vi "CODMn报警信息存储.vi"(8 "error in (no error)":errorcluster, 11 "data in":T1) -> (0 "error out":errorcluster)   [LabVIEW 2016, in "斯坦道CODMn.lvlib"]
uses:
  <vilib>/addons/database/Auxilliary.llb/DB Tools Transaction.ctl
  <vilib>/addons/database/Auxilliary.llb/DB Tools Isolation Level.ctl
  <vilib>/addons/database/Auxilliary.llb/DB Tools Column Info.ctl
  <vilib>/addons/database/Auxilliary.llb/DB Tools DataTypes.ctl
  <vilib>/addons/database/Auxilliary.llb/DB Tools Parameter Info.ctl
  <vilib>/addons/database/Auxilliary.llb/DB Tools Parameter Dir.ctl
  <vilib>/addons/database/Connection.llb/DB Tools Open Connec (String).vi
  <vilib>/addons/database/Connection.llb/Conn Transaction.vi
  <vilib>/addons/database/Connection.llb/Conn Execute.vi
  <vilib>/addons/database/Recordset.llb/Rec Destroy - Connection.vi
  <vilib>/addons/database/Command.llb/Cmd Set Parameter Value (C).vi
  <vilib>/addons/database/Auxilliary.llb/DB Tools Format Datetime String (Time Stamp).vi
  <vilib>/addons/database/Command.llb/Cmd Execute.vi
  <vilib>/addons/database/Recordset.llb/Rec Destroy - Command.vi
  <vilib>/addons/database/Command.llb/Cmd Delete.vi
  <vilib>/addons/database/NI_Database_API.lvlib
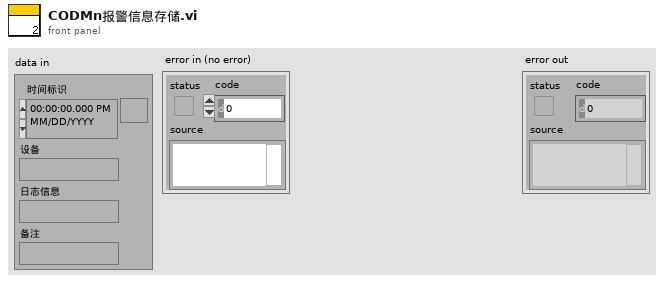
[diagram p1: front panel]
types:
  T1 = cluster{"时间标识":timestamp, "设备":string, "日志信息":string, "备注":string}
  T2 = typedef "NI_Database_API.lvlib/DB Tools Column Info.ctl" = cluster{"column name":string, "data type":T3, "size":i32, "allow null?":bool}
  T3 = typedef "NI_Database_API.lvlib/DB Tools DataTypes.ctl" = enum16{"String", "Long (I32)", "Single (SGL)", "Double (DBL)", "Date/Time", "Binary"}
  T4 = typedef "NI_Database_API.lvlib/DB Tools Isolation Level.ctl" = enum16{"chaos", "read uncommitted", "read committed", "repeatable read", "serializable"}
  T5 = typedef "NI_Database_API.lvlib/DB Tools Transaction.ctl" = enum16{"begin", "commit", "rollback"}
  T6 = typedef "NI_Database_API.lvlib/Conn ObjectReference.ctl" = refnum<k1>
  T7 = typedef "NI_Database_API.lvlib/DB Tools Parameter Info.ctl" = cluster{"parameter name":string, "type":T3, "direction":T8, "value":variant}
  T8 = typedef "NI_Database_API.lvlib/DB Tools Parameter Dir.ctl" = enum32{"Input", "Output", "Input/Output", "Return Value"}
  T9 = typedef "NI_Database_API.lvlib/Rec ObjectReference.ctl" = refnum<k1>
  T10 = typedef "NI_Database_API.lvlib/Cmd ObjectReference.ctl" = refnum<k1>
  T11 = typedef "NI_Database_API.lvlib/Cmd-Rec Object Reference.ctl" = refnum<k1>
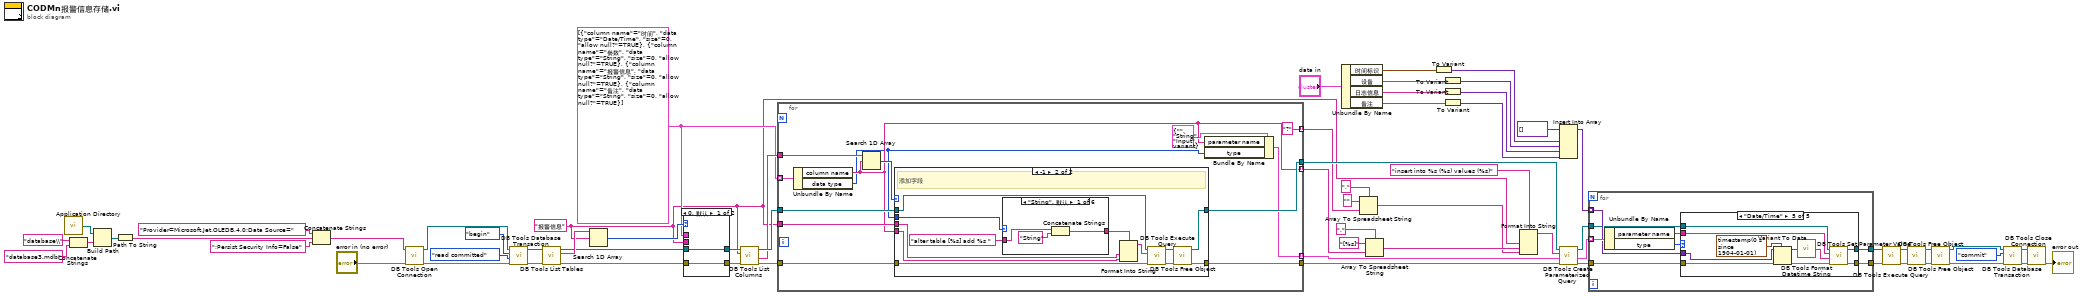
[diagram p0: block diagram]
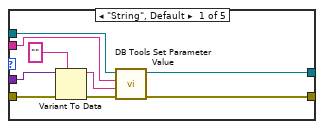
[diagram p2: hidden frame]
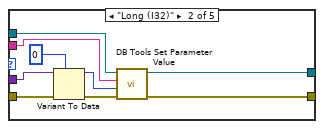
[diagram p3: hidden frame]
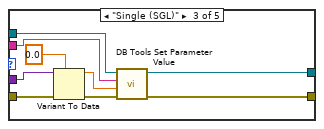
[diagram p4: hidden frame]
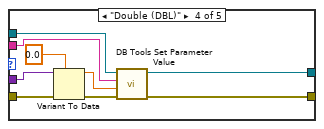
[diagram p5: hidden frame]
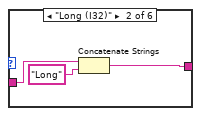
[diagram p7: hidden frame]
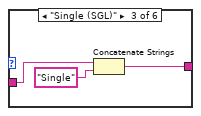
[diagram p8: hidden frame]
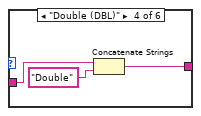
[diagram p9: hidden frame]
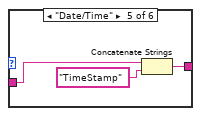
[diagram p10: hidden frame]
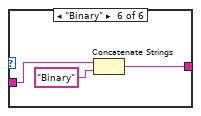
[diagram p11: hidden frame]
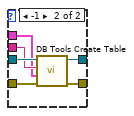
[diagram p12: hidden frame]
diagram:
  w45 = T2[] [{"column name"="时间", "data type"=enum."Date/Time", "size"=0, "allow null?"=TRUE}, {"column name"="参数", "data type"=enum."String", "size"=0, "allow null?"=TRUE}, {"column name"="报警信息", "data type"=enum."String", "size"=0, "allow null?"=TRUE}, {"column name"="备注", "data type"=enum."String", "size"=0, "allow null?"=TRUE}] ("column information")
  w38 = "报警信息"
  n1 = call <vilib>:"Application Directory.vi"() -> ("Application Directory"=w1:path)
  n2 = Concatenate Strings("database\\" ("condition"), "database3.mdb" ("database")) -> (w59:string)
  n3 = Build Path(base path=w1, name or relative path=w59) -> (appended path=w64:path)
  n4 = Path To String(path=w64) -> (string=w63:string)
  n5 = Concatenate Strings("Provider=Microsoft.Jet.OLEDB.4.0;Data Source=" ("condition"), w63, ";Persist Security Info=False" ("condition")) -> (w61:string)
  n6 = call-poly <vilib>:"DB Tools Open Connection.vi"("error in (no error)"="error in (no error)", "connection information"=w61) -> ("error out"=w3:errorcluster, "connection reference"=w5:T6)  [unwired: 6 in]
  n7 = call-poly <vilib>:"DB Tools Database Transaction.vi"("error in (no error)"=w3, "isolation level (chaos)"=DB_Tools_Isolation_Level."read committed", "operation (begin)"=DB_Tools_Transaction."begin", "connection reference"=w5) -> ("error out"=w2:errorcluster, "connection reference out"=w4:T6)  [unwired: 2 in]
  n8 = call <vilib>:"DB Tools List Tables.vi"("error in (no error)"=w2, "connection reference"=w4) -> ("error out"=w49:errorcluster, "tables"=w52:string[], "connection reference out"=w50:T6)  [unwired: 3 in]
  n9 = Search 1D Array(1D array=w52, element=w38) -> (index of element=w51:i32)  [unwired: 1 in]
  n10 = case shown="0, 默认" w51 {
    tunnel: w50 -> [w68 w74]
    tunnel: w49 -> [w67 w73]
    tunnel: w38 -> [_ w72]
    tunnel: w45 -> [_ w71]
    tunnel: [w68 w70] -> w44
    tunnel: [w67 w69] -> w43
    frame 0, Default {
    }
    frame -1 {
      n11 = call <vilib>:"DB Tools Create Table.vi"("error in (no error)"=w73, "column information"=w71, "table"=w72, "connection reference"=w74) -> ("error out"=w69:errorcluster, "connection reference out"=w70:T6)  [unwired: 4 in]
    }
  }
  n12 = call <vilib>:"DB Tools List Columns.vi"("error in (no error)"=w43, "table"=w38, "connection reference"=w44) -> ("error out"=w46:errorcluster, "columns"=w47:string[], "connection reference out"=w48:T6)  [unwired: 1 in, 1 out]
  n13 = for {
    tunnel: w48 -> [w85]
    tunnel: w47 -> [w87]
    tunnel: w46 -> [w84]
    tunnel: [w83] -> w42
    tunnel: [w82] -> w41
    tunnel: w38 -> [w81]
    tunnel: w45 -> [w80] mode=indexing
    tunnel: [w78] -> w40 mode=indexing
    tunnel: [w77] -> w33 mode=indexing
    tunnel: ["?"] -> w31 mode=indexing
    n14 = Unbundle By Name(w80) -> ("column name"=w77:string, "data type"=w75:T3)
    n15 = Search 1D Array(1D array=w87, element=w77) -> (index of element=w86:i32)  [unwired: 1 in]
    n16 = case shown="-1" w86 {
      tunnel: [w89 w98] -> w82
      tunnel: [w88 w97] -> w83
      tunnel: w85 -> [w89 w96]
      tunnel: w77 -> [_ w95]
      tunnel: w84 -> [w88 w94]
      tunnel: w81 -> [_ w93]
      tunnel: w75 -> [_ w91]
      frame 0, Default {
      }
      frame -1 {
        # "添加字段"
        n17 = case shown="\"String\", 默认" w91 {
          tunnel: "alter table [%s] add %s " -> [w104 w107 w110 w113 w116 w119]
          tunnel: [w103 w106 w109 w112 w115 w118] -> w90
          frame "String", Default {
            n18 = Concatenate Strings(w104, "String" ("字符串")) -> (w103:string)
          }
          frame "Long (I32)" {
            n19 = Concatenate Strings(w107, "Long" ("字符串")) -> (w106:string)
          }
          frame "Single (SGL)" {
            n20 = Concatenate Strings(w110, "Single" ("字符串")) -> (w109:string)
          }
          frame "Double (DBL)" {
            n21 = Concatenate Strings(w113, "Double" ("字符串")) -> (w112:string)
          }
          frame "Date/Time" {
            n22 = Concatenate Strings(w116, "TimeStamp" ("字符串")) -> (w115:string)
          }
          frame "Binary" {
            n23 = Concatenate Strings(w119, "Binary" ("字符串")) -> (w118:string)
          }
        }
        n24 = Format Into String(format string=w90, w93, w95) -> (resulting string=w99:string)  [unwired: 2 in, 1 out]
        n25 = call-poly <vilib>:"DB Tools Execute Query.vi"("error in (no error)"=w94, "SQL query"=w99, "connection reference"=w96) -> ("error out"=w100:errorcluster, "recordset reference"=w101:T9)  [unwired: 5 in]
        n26 = call-poly <vilib>:"DB Tools Free Object.vi"("error in (no error)"=w100, "recordset reference"=w101) -> ("error out"=w97:errorcluster, "connection reference"=w98:T6)  [unwired: 8 in]
      }
    }
    n27 = Bundle By Name(cluster=T7 {"parameter name"="", "type"=enum."String", "direction"=enum."Input", "value"=variant} ("parameter information"), "parameter name"=w77, "type"=w75) -> (w78:T7)
  }
  n28 = Unbundle By Name("data in") -> ("时间标识"=w25:timestamp, "设备"=w22:string, "日志信息"=w23:string, "备注"=w24:string)
  n29 = Array To Spreadsheet String(delimiter (Tab)="," ("分隔符(Tab)"), array=w31, 3:"" ("格式字符串")) -> (spreadsheet string=w30:string)
  n30 = Array To Spreadsheet String(delimiter (Tab)="," ("分隔符(Tab)"), array=w33, 3:"[%s]" ("格式字符串")) -> (spreadsheet string=w32:string)
  n31 = To Variant(anything=w25) -> (Variant=w20:variant)
  n32 = To Variant(anything=w22) -> (Variant=w19:variant)
  n33 = To Variant(anything=w23) -> (Variant=w18:variant)
  n34 = To Variant(anything=w24) -> (Variant=w17:variant)
  n35 = Format Into String(format string="insert into %s (%s) values (%s)" ("格式字符串"), w38, w32, w30) -> (resulting string=w29:string)  [unwired: 2 in, 1 out]
  n36 = Insert Into Array(array=variant[] [], new element #1=w20, new element #2=w19, new element #3=w18, new element #4=w17) -> (w16:variant[])  [unwired: 1 in]
  n37 = call <vilib>:"DB Tools Create Parameterized Query.vi"("error in (no error)"=w42, "parameters"=w40, "SQL query"=w29, "connection reference"=w41) -> ("error out"=w27:errorcluster, "parameters out"=w26:T7[], "command reference"=w28:T10)  [unwired: 3 in]
  n38 = for {
    tunnel: w28 -> [w124]
    tunnel: w27 -> [w122]
    tunnel: w26 -> [w127] mode=indexing
    tunnel: w16 -> [w125] mode=indexing
    tunnel: [w121] -> w15
    tunnel: [w120] -> w14
    n39 = Unbundle By Name(w127) -> ("parameter name"=w123:string, "type"=w126:T3)
    n40 = case shown="\"Date/Time\"" w126 {
      tunnel: w125 -> [w131 w139 w146 w156 w173]
      tunnel: w124 -> [w134 w143 w150 w160 w171]
      tunnel: w123 -> [w133 w142 w149 w155 w170]
      tunnel: w122 -> [w128 w137 w147 w157 w168]
      tunnel: [w130 w141 w151 w159 w167] -> w121
      tunnel: [w129 w140 w148 w158 w166] -> w120
      frame "String", Default {
        n41 = Variant To Data(error in=w128, type="", Variant=w131) -> (data=w132:string, error out=w136:errorcluster)
        n42 = call-poly <vilib>:"DB Tools Set Parameter Value.vi"("error in (no error)"=w136, "value"=w132, "parameter index"=w133, "command reference"=w134) -> ("error out"=w129:errorcluster, "command reference out"=w130:T10)  [unwired: 4 in]
      }
      frame "Long (I32)" {
        n43 = Variant To Data(error in=w137, type=0, Variant=w139) -> (data=w144:i32, error out=w145:errorcluster)
        n44 = call-poly <vilib>:"DB Tools Set Parameter Value.vi"("error in (no error)"=w145, "value"=w144, "parameter index"=w142, "command reference"=w143) -> ("error out"=w140:errorcluster, "command reference out"=w141:T10)  [unwired: 4 in]
      }
      frame "Single (SGL)" {
        n45 = Variant To Data(error in=w147, type=sgl 0.0, Variant=w146) -> (data=w153:sgl, error out=w154:errorcluster)
        n46 = call-poly <vilib>:"DB Tools Set Parameter Value.vi"("error in (no error)"=w154, "value"=w153, "parameter index"=w149, "command reference"=w150) -> ("error out"=w148:errorcluster, "command reference out"=w151:T10)  [unwired: 4 in]
      }
      frame "Double (DBL)" {
        n47 = Variant To Data(error in=w157, type=0.0, Variant=w156) -> (data=w162:dbl, error out=w163:errorcluster)
        n48 = call-poly <vilib>:"DB Tools Set Parameter Value.vi"("error in (no error)"=w163, "value"=w162, "parameter index"=w155, "command reference"=w160) -> ("error out"=w158:errorcluster, "command reference out"=w159:T10)  [unwired: 4 in]
      }
      frame "Date/Time" {
        n49 = Variant To Data(error in=w168, type=timestamp(0 s since 1904-01-01) ("时间标识"), Variant=w173) -> (data=w165:timestamp, error out=w169:errorcluster)
        n50 = call-poly <vilib>:"DB Tools Format Datetime String.vi"("time stamp"=w165) -> ("date/time string"=w164:string)
        n51 = call-poly <vilib>:"DB Tools Set Parameter Value.vi"("error in (no error)"=w169, "value"=w164, "parameter index"=w170, "command reference"=w171) -> ("error out"=w166:errorcluster, "command reference out"=w167:T10)  [unwired: 4 in]
      }
    }
  }
  n52 = call-poly <vilib>:"DB Tools Execute Query.vi"("error in (no error)"=w14, "command reference"=w15) -> ("error out"=w12:errorcluster, "command-recordset reference"=w13:T11)  [unwired: 6 in]
  n53 = call-poly <vilib>:"DB Tools Free Object.vi"("error in (no error)"=w12, "command-recordset reference"=w13) -> ("error out"=w10:errorcluster, "command reference"=w11:T10)  [unwired: 8 in]
  n54 = call-poly <vilib>:"DB Tools Free Object.vi"("error in (no error)"=w10, "command reference"=w11) -> ("error out"=w6:errorcluster, "connection reference"=w7:T6)  [unwired: 8 in]
  n55 = call-poly <vilib>:"DB Tools Database Transaction.vi"("error in (no error)"=w6, "operation (begin)"=DB_Tools_Transaction."commit", "connection reference"=w7) -> ("error out"=w8:errorcluster, "connection reference out"=w9:T6)  [unwired: 3 in]
  n56 = call <vilib>:"DB Tools Close Connection.vi"("error in (no error)"=w8, "connection reference"=w9) -> ("error out"=→"error out":errorcluster)  [unwired: 5 in]
